vi "SPCUpdateStatus.vi"(0 "Status":u16(ring) items=["offline", "online", "busy"]) -> ()   [LabVIEW 2009]
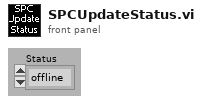
[diagram p1: front panel]
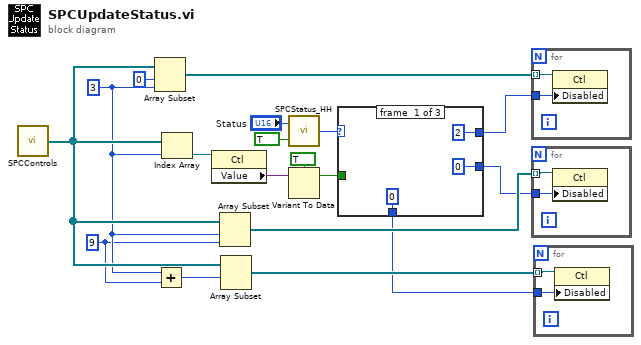
[diagram p0: block diagram]
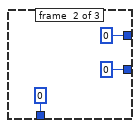
[diagram p2: hidden frame]
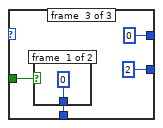
[diagram p3: hidden frame]
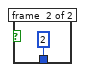
[diagram p4: hidden frame]
diagram:
  w5 = 3 ("index")
  w1 = 9 ("length")
  n1 = call "SPCControls.vi"() -> ("Control References (output)"=w7:refnum<vi>[])  [unwired: 2 in]
  n2 = Array Subset(array=w7, index=0, length=w5) -> (w4:refnum<vi>[])
  n3 = Add(x=w5, y=w1) -> (x+y=w9:i32)
  n4 = Index Array(array=w7, index=w5) -> (element=w8:refnum<vi>)
  n5 = property class="Ctl"(reference=w8) -> ("Value"=w12:variant)  [unwired: 1 in, 2 out]
  n6 = Array Subset(array=w7, index=w5, length=w1) -> (w18:refnum<vi>[])
  n7 = Array Subset(array=w7, index=w9) -> (w14:refnum<vi>[])  [unwired: 1 in]
  n8 = call "SPCStatus_HH.vi"("Set/Get"=TRUE, "Status (input)"="Status") -> ("Status (output)"=w15:enum16{"offline", "online", "busy"})
  n9 = Variant To Data(Variant=w12, type=TRUE ("Set/Get")) -> (data=w13:bool)  [unwired: 1 in, 1 out]
  n10 = case shown="\"busy\"" w15 {
    tunnel: [u8 2 ("Disabled") u8 0 ("Disabled") u8 0 ("Disabled")] -> w3
    tunnel: [u8 0 ("Disabled") u8 0 ("Disabled") u8 2 ("Disabled")] -> w2
    tunnel: w13 -> [_ _ w26]
    tunnel: [u8 0 ("Disabled") u8 0 ("Disabled") w25] -> w10
    frame #0 {
    }
    frame #1 {
    }
    frame #2 {
      n11 = case shown="False" w26 {
        tunnel: [u8 0 ("Disabled") u8 2 ("Disabled")] -> w25
        frame #0 {
        }
        frame #1 {
        }
      }
    }
  }
  n12 = for {
    tunnel: w4 -> [w32] mode=indexing
    tunnel: w3 -> [w31]
    n13 = property class="Ctl"(reference=w32, "Disabled"=w31) -> ()  [unwired: 1 in, 2 out]
  }
  n14 = for {
    tunnel: w18 -> [w34] mode=indexing
    tunnel: w2 -> [w33]
    n15 = property class="Ctl"(reference=w34, "Disabled"=w33) -> ()  [unwired: 1 in, 2 out]
  }
  n16 = for {
    tunnel: w14 -> [w36] mode=indexing
    tunnel: w10 -> [w35]
    n17 = property class="Ctl"(reference=w36, "Disabled"=w35) -> ()  [unwired: 1 in, 2 out]
  }
